vi "uObserver_Get_BrokerIsOwner.vi"(8 "error in (no error)":errorcluster, 11 "uObserver in":refnum<class "uObserver.lvclass">) -> (0 "error out":errorcluster, 2 "Broker.IsOwner?":bool, 3 "uObserver out":refnum<class "uObserver.lvclass">)   [LabVIEW 2023, in "uFramework_pack_uActor.lvlib" / "uObserver.lvclass"]
doc: "Use to check if this observer owns its own broker."
uses:
  uObserver.lvclass
  uObserver.lvclass/uObserver.ctl
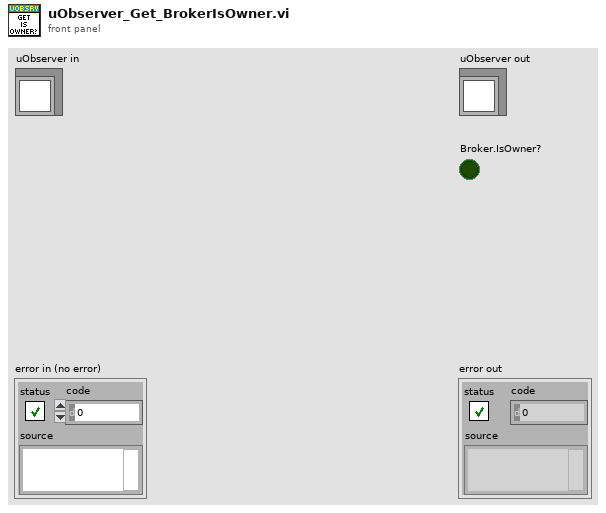
[diagram p1: front panel]
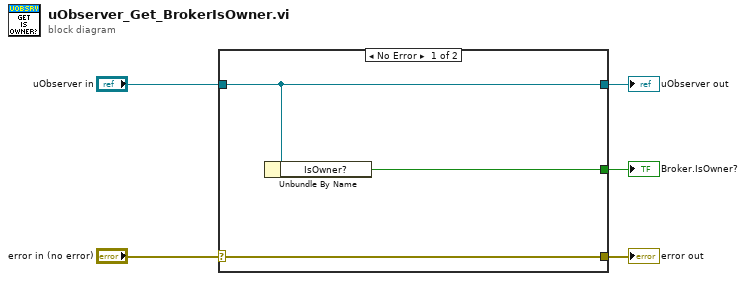
[diagram p0: block diagram]
diagram:
  n1 = case shown="No Error" "error in (no error)" {
    selector: "error in (no error)" -> [w8 w9]
    tunnel: [w8 w9] -> w4
    tunnel: [w7 w10] -> w2
    tunnel: "uObserver in" -> [w7 w10]
    tunnel: [w6 _] -> w1
    frame No Error {
      n2 = Unbundle By Name(w7) -> ("IsOwner?"=w6:bool)
    }
    frame Error {
    }
  }
  "error out" <- w4
  "uObserver out" <- w2
  "Broker.IsOwner?" <- w1
